vi "Basic Test Compile, Proof of Concept.vi"() -> ()   [LabVIEW 2009]
uses:
  Motor Control Global.vi
  <vilib>/Platform/TimedLoop/XDataNode/XDataNode.xnode
  <vilib>/Platform/TimedLoop/XDataNode/loadlvalarms.vi
  <vilib>/Platform/TimedLoop/XDataNode/timing_clust.ctl
  <vilib>/Platform/TimedLoop/XDataNode/nitl_modes.ctl
  <vilib>/Platform/TimedLoop/XDataNode/wakeup.ctl
  <vilib>/Platform/TimedLoop/XDataNode/XDNodeRunTimeDep.lvlib
panel:
  out "Tick Count Differencce":u32
  out "Tick Count(Ticks) 2":u32 caption="Tick Count(Ticks)"
  out "Tick Count(Ticks)":u32
  in  "Single Cycle":bool
  out "Multiplication Result":fxp<+/-,18,1> format="%.18g"
  out "i 3":i32
  out "i 2":i32
  out "i 1":i32
  out "in wait":bool=TRUE
  in  "Restart":bool
  in  "Input F":fxp<+/-,18,1>
  in  "Input E":fxp<+/-,18,1>
  out "Multiplication Result 8 iterations of madness":fxp<+/-,18,1> format="%.18g"
  in  "Input D":fxp<+/-,18,1>
  in  "Input C":fxp<+/-,18,1>
  out "Multiplication Result C^2^15 * D^2^15":fxp<+/-,18,1> format="%.18g"
  in  "stop":bool
  out "Multiplication Result A^60*B":fxp<+/-,18,1> format="%.18g"
  in  "Input A":fxp<+/-,18,1>
  in  "Input B":fxp<+/-,18,1>
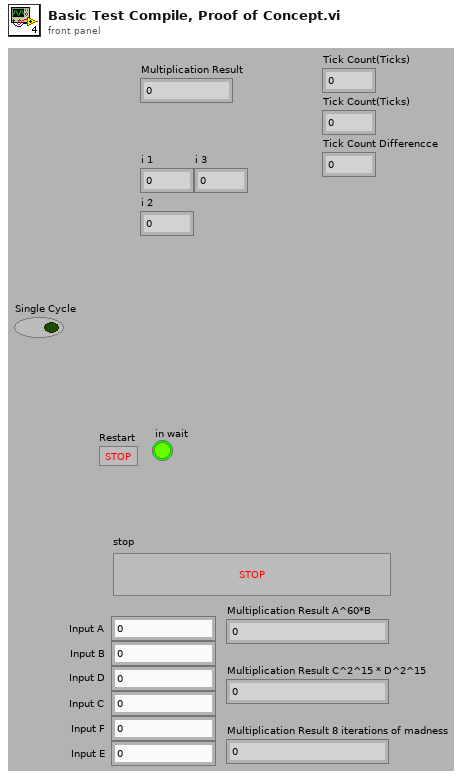
[diagram p1: front panel]
types:
  T1 = typedef "XDNodeRunTimeDep.lvlib/timing_clust.ctl" = cluster{"Expected End [f-1]":u64, "Actual End [f-1]":u64, "Finished Late? [f-1]":bool, "Expected End [i-1]":u64, "Actual End [i-1]":u64, "Finished Late? [i-1]":bool, "Expected Start [i]":u64, "Actual Start [i]":u64, "Expected Start [f]":u64, "Actual Start [f]":u64, "Source Name":string, "Structure Name":string, "Period":i64, "Deadline":i64, "Offset":i64, "Start":i64, "Priority":i32, "Timeout":i32, "Mode":T2, "Wakeup Reason":T3, "Error":errorcluster, "Source Type":string, "Secondary Source Type":string, "Global End Time":u64, "Global Start Time":u64, "Frame Duration":u64, "Iteration Duration":u64, "Assigned CPU":i32, "I/O Scan Engine Mode":u32}
  T2 = typedef "XDNodeRunTimeDep.lvlib/nitl_modes.ctl" = enum32{"No Change", "Process missed periods, maintain original phase", "Discard missed periods, maintain original phase", "Process missed periods, ignore original phase", "Discard missed periods, ignore original phase"}
  T3 = typedef "XDNodeRunTimeDep.lvlib/wakeup.ctl" = enum32{"Normal", "Aborted", "Asynchronous wakeup", "Timing source error", "Timed loop error", "Timeout"}
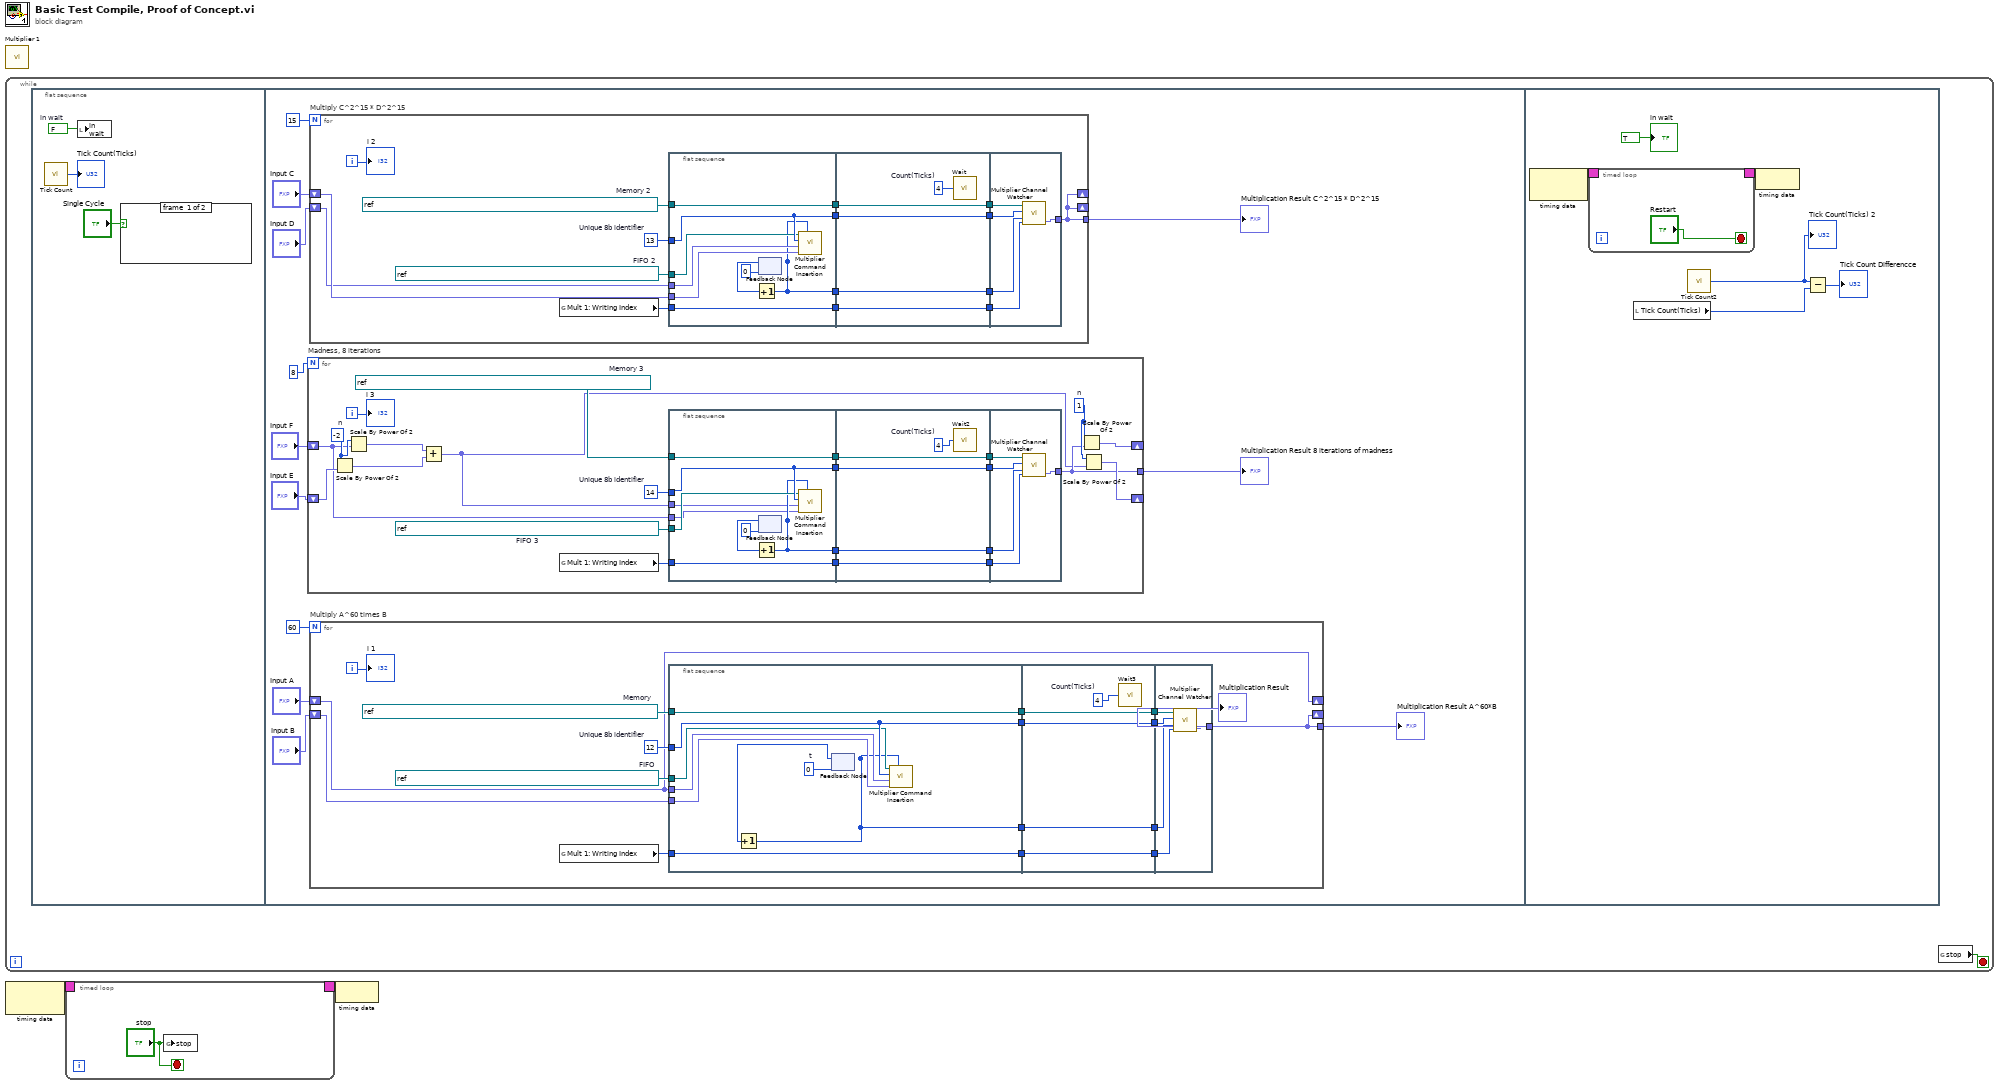
[diagram p0: block diagram]
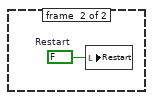
[diagram p2: hidden frame]
diagram:
  n1 = call "Multiplier 1.vi"() -> ()  [unwired: 1 in]
  n2 = while {
    stop <- w3 stop-if-true
    n3 = flat-sequence {
      frame #0 {
        w6 = FALSE  # in wait
        n4 = call "Tick Count"() -> ("Tick Count(Ticks)"=→"Tick Count(Ticks)":u32)
        n5 = local write "in wait"(w6) -> ()
        n6 = case shown="True" "Single Cycle" {
          frame #0 {
          }
          frame #1 {
            w7 = FALSE  # Restart
            n7 = local write "Restart"(w7) -> ()
          }
        }
      }
      frame #1 {
        n8 = for "Madness, 8 iterations" {
          N: 8 -> [_]
          shift-right: [w28] -> _
          shift-left: "Input F" -> [w20]
          shift-right: [w27] -> _
          shift-left: "Input E" -> [w38]
          tunnel: [w22] -> w8
          i -> [w37]
          w26 = 1  # n
          w25 = -2  # n
          w42 = refnum<k21> "Multiplier 1 FIFO In :  [8b Idendifier; 20b args; 18b fxp ; 18b fxp]"  # FIFO 3
          w41 = refnum<k21> "Multiplier 1 Block Memory Out : [8b Identifier; 6b args; 18b fxp output]"  # Memory 3
          w40 = u8 14  # Unique 8b identifier
          n9 = Scale By Power Of 2(n=w25, x=w38) -> (x*2^n=w23:fxp<+/-,18,1>)
          n10 = Scale By Power Of 2(n=w25, x=w20) -> (x*2^n=w24:fxp<+/-,18,1>)
          n11 = Add(x=w24, y=w23) -> (x+y=w21:fxp<+/-,18,1>)
          n12 = global read "Motor Control Global.vi" "Mult 1: Writing Index"() -> (w39:u32)
          n13 = flat-sequence {
            tunnel: [w51] -> w36
            tunnel: [w50] -> w34
            tunnel: [w46] -> w32
            tunnel: [w47] -> w30
            tunnel: w40 -> [w51]
            tunnel: w42 -> [w49]
            tunnel: w41 -> [w50]
            tunnel: w39 -> [w46]
            tunnel: w21 -> [w44]
            tunnel: w20 -> [w43]
            tunnel: w36 -> [w56]
            tunnel: [w56] -> w35
            tunnel: w34 -> [w55]
            tunnel: [w55] -> w33
            tunnel: w32 -> [w54]
            tunnel: [w54] -> w31
            tunnel: w30 -> [w53]
            tunnel: [w53] -> w29
            tunnel: w35 -> [w61]
            tunnel: w33 -> [w60]
            tunnel: w31 -> [w59]
            tunnel: w29 -> [w58]
            tunnel: [w57] -> w22
            frame #0 {
              n14 = feedback #1(u8 0) -> (w48:u8)
              n15 = Increment(x=w48) -> (x+1=w47:u8)
              n16 = call "Multiplier Command Insertion.vi"("Counter Descriminator"=w47, "Input B"=w43, "Input A"=w44, "Channel Identifier"=w51, "FIFO"=w49) -> ()  [unwired: 6 in, 1 out]
            }
            frame #1 {
              w52 = u32 4  # Count(Ticks)
              n17 = call "Wait2"("Count(Ticks)"=w52) -> ()  [unwired: 1 out]
            }
            frame #2 {
              n18 = call "Multiplier Channel Watcher.vi"("Block Memory"=w60, "Watched Channel"=w61, "Count to match"=w58, "Writing Index Start"=w59) -> ("Multiplication Result"=w57:fxp<+/-,18,1>)  [unwired: 1 in, 2 out]
            }
          }
          n19 = Scale By Power Of 2(n=w26, x=w22) -> (x*2^n=w28:fxp<+/-,18,1>)
          n20 = Scale By Power Of 2(n=w26, x=w21) -> (x*2^n=w27:fxp<+/-,18,1>)
          "i 3" <- w37
        }
        "Multiplication Result 8 iterations of madness" <- w8
        n21 = for "Multiply C^2^15 * D^2^15" {
          N: 15 -> [_]
          shift-right: [w71] -> _
          shift-left: "Input D" -> [w72]
          shift-right: [w71] -> _
          shift-left: "Input C" -> [w73]
          tunnel: [w71] -> w15
          i -> [w70]
          w77 = refnum<k21> "Multiplier 1 FIFO In :  [8b Idendifier; 20b args; 18b fxp ; 18b fxp]"  # FIFO 2
          w76 = refnum<k21> "Multiplier 1 Block Memory Out : [8b Identifier; 6b args; 18b fxp output]"  # Memory 2
          w75 = u8 13  # Unique 8b identifier
          n22 = global read "Motor Control Global.vi" "Mult 1: Writing Index"() -> (w74:u32)
          n23 = flat-sequence {
            tunnel: [w86] -> w69
            tunnel: [w85] -> w67
            tunnel: [w79] -> w65
            tunnel: [w80] -> w63
            tunnel: w72 -> [w83]
            tunnel: w73 -> [w82]
            tunnel: w75 -> [w86]
            tunnel: w77 -> [w84]
            tunnel: w76 -> [w85]
            tunnel: w74 -> [w79]
            tunnel: w69 -> [w91]
            tunnel: [w91] -> w68
            tunnel: w67 -> [w90]
            tunnel: [w90] -> w66
            tunnel: w65 -> [w89]
            tunnel: [w89] -> w64
            tunnel: w63 -> [w88]
            tunnel: [w88] -> w62
            tunnel: w68 -> [w96]
            tunnel: w66 -> [w95]
            tunnel: w64 -> [w94]
            tunnel: w62 -> [w93]
            tunnel: [w92] -> w71
            frame #0 {
              n24 = feedback #2(u8 0) -> (w81:u8)
              n25 = Increment(x=w81) -> (x+1=w80:u8)
              n26 = call "Multiplier Command Insertion.vi"("Counter Descriminator"=w80, "Input B"=w82, "Input A"=w83, "Channel Identifier"=w86, "FIFO"=w84) -> ()  [unwired: 6 in, 1 out]
            }
            frame #1 {
              w87 = u32 4  # Count(Ticks)
              n27 = call "Wait"("Count(Ticks)"=w87) -> ()  [unwired: 1 out]
            }
            frame #2 {
              n28 = call "Multiplier Channel Watcher.vi"("Block Memory"=w95, "Watched Channel"=w96, "Count to match"=w93, "Writing Index Start"=w94) -> ("Multiplication Result"=w92:fxp<+/-,18,1>)  [unwired: 1 in, 2 out]
            }
          }
          "i 2" <- w70
        }
        "Multiplication Result C^2^15 * D^2^15" <- w15
        n29 = for "Multiply A^60 times B" {
          N: 60 -> [_]
          shift-right: [w107] -> _
          shift-left: "Input A" -> [w107]
          shift-right: [w106] -> _
          shift-left: "Input B" -> [w108]
          tunnel: [w106] -> w16
          i -> [w105]
          w111 = refnum<k21> "Multiplier 1 Block Memory Out : [8b Identifier; 6b args; 18b fxp output]"  # Memory
          w112 = refnum<k21> "Multiplier 1 FIFO In :  [8b Idendifier; 20b args; 18b fxp ; 18b fxp]"  # FIFO
          w110 = u8 12  # Unique 8b identifier
          n30 = global read "Motor Control Global.vi" "Mult 1: Writing Index"() -> (w109:u32)
          n31 = flat-sequence {
            tunnel: [w121] -> w104
            tunnel: [w120] -> w102
            tunnel: [w116] -> w100
            tunnel: [w113] -> w98
            tunnel: w107 -> [w118]
            tunnel: w108 -> [w117]
            tunnel: w110 -> [w121]
            tunnel: w112 -> [w119]
            tunnel: w111 -> [w120]
            tunnel: w109 -> [w116]
            tunnel: w104 -> [w126]
            tunnel: [w126] -> w103
            tunnel: w102 -> [w125]
            tunnel: [w125] -> w101
            tunnel: w100 -> [w124]
            tunnel: [w124] -> w99
            tunnel: w98 -> [w123]
            tunnel: [w123] -> w97
            tunnel: w103 -> [w131]
            tunnel: w101 -> [w130]
            tunnel: w99 -> [w129]
            tunnel: w97 -> [w128]
            tunnel: [w127] -> w106
            frame #0 {
              w114 = u8 0  # t
              n32 = feedback #3(w114) -> (w115:u8)
              n33 = Increment(x=w115) -> (x+1=w113:u8)
              n34 = call "Multiplier Command Insertion.vi"("Counter Descriminator"=w113, "Input B"=w117, "Input A"=w118, "Channel Identifier"=w121, "FIFO"=w119) -> ()  [unwired: 6 in, 1 out]
            }
            frame #1 {
              w122 = u32 4  # Count(Ticks)
              n35 = call "Wait3"("Count(Ticks)"=w122) -> ()  [unwired: 1 out]
            }
            frame #2 {
              n36 = call "Multiplier Channel Watcher.vi"("Block Memory"=w130, "Watched Channel"=w131, "Count to match"=w128, "Writing Index Start"=w129) -> ("Multiplication Result"=w127:fxp<+/-,18,1>)  [unwired: 1 in, 2 out]
            }
          }
          "i 1" <- w105
          "Multiplication Result" <- w106
        }
        "Multiplication Result A^60*B" <- w16
      }
      frame #2 {
        n37 = node-c288() -> (w136:T1)  [unwired: 1 in]
        n38 = timed-loop {
          timing: w136 -> [_]
          timing-out: [_] -> w135
          stop <- "Restart" stop-if-true
        }
        n39 = local read "Tick Count(Ticks)"() -> (w137:u32)
        n40 = call "Tick Count2"() -> ("Tick Count(Ticks)"=w133:u32)
        "Tick Count(Ticks) 2" <- w133
        n41 = node-c288(w135) -> ()
        n42 = Subtract(x=w133, y=w137) -> (x-y=→"Tick Count Differencce":u32)
        "in wait" <- TRUE
      }
    }
    n43 = global read "Motor Control Global.vi" "stop"() -> (w3:bool)
  }
  n44 = node-c288() -> (w2:T1)  [unwired: 1 in]
  n45 = timed-loop {
    timing: w2 -> [_]
    timing-out: [_] -> w1
    stop <- "stop" stop-if-true
    n46 = global write "Motor Control Global.vi" "stop"("stop") -> ()
  }
  n47 = node-c288(w1) -> ()
